vi "Constantes.vi"() -> ()   [LabVIEW 2016]
panel:
  in  "VisionOverlayIndex Max":dbl=5.0
  in  "Nomber of reload steps":dbl=10.0
  in  "Joystick DeadZone":dbl(slide)=0.031914893617021274 scale=0.0..1.0
  in  "Input Y Factor":dbl(slide)=0.5 scale=0.0..1.0
  in  "Input X Factor":dbl(slide)=0.5 scale=0.0..1.0
  in  "Block forward when distance to a wall is under":dbl=7.0
  # "Teleop Driving"
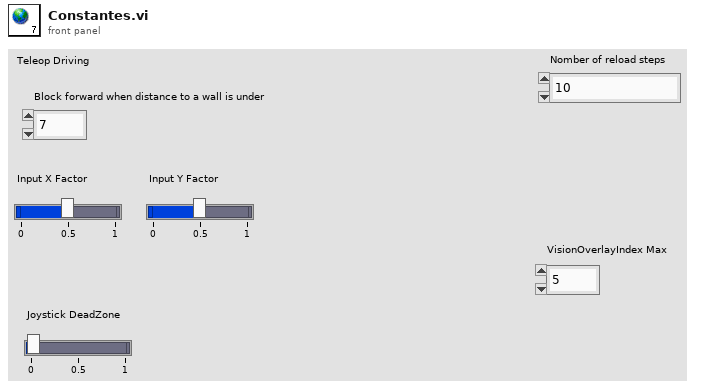
[diagram p1: front panel]
diagram:
